vi "Cable Length Param.vi"(8 "error constant":errorcluster) -> (0 "error out":errorcluster, 2 "Cable Length Param":string)   [LabVIEW 2017]
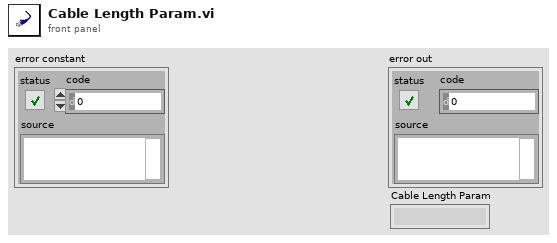
[diagram p1: front panel]
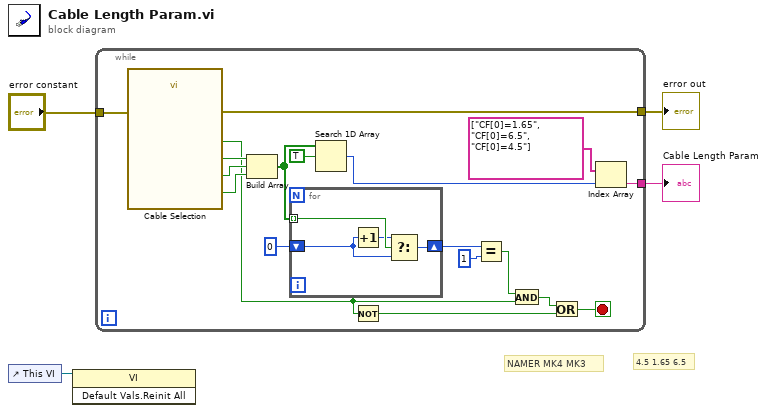
[diagram p0: block diagram]
diagram:
  # "4.5 1.65 6.5"
  # "NAMER MK4 MK3"
  n1 = control-ref of="This VI"() -> (w1:refnum<vi>)
  n2 = invoke class="VI" method="Default Vals.Reinit All"(reference=w1) -> ()  [unwired: 2 in, 3 out]
  n3 = while {
    tunnel: "error constant" -> [w20]
    tunnel: [w19] -> w3
    tunnel: [w9] -> w2
    stop <- w8 stop-if-true
    n4 = call "Cable Selection"("error in (no error)"=w20) -> ("NAMER"=w12:bool, "MK3"=w22:bool, "MK4"=w13:bool, "OK"=w5:bool, "error out"=w19:errorcluster)  [unwired: 14 in]
    n5 = Build Array(w13, w22, w12) -> (w18:bool[])
    n6 = for {
      tunnel: w18 -> [w26] mode=indexing
      shift-right: [w24] -> w16
      shift-left: 0 -> [w23]
      n7 = Increment(x=w23) -> (x+1=w25:i32)
      n8 = Select(t=w25, s=w26, f=w23) -> (s? t:f=w24:i32)
    }
    n9 = Search 1D Array(1D array=w18, element=TRUE) -> (index of element=w10:i32)  [unwired: 1 in]
    n10 = Not(x=w5) -> (.not. x?=w6:bool)
    n11 = Equal?(x=w16, y=1) -> (x = y?=w14:bool)
    n12 = And(x=w14, y=w5) -> (x .and. y?=w7:bool)
    n13 = Or(x=w7, y=w6) -> (x .or. y?=w8:bool)
    n14 = Index Array(array=string[] ["CF[0]=1.65", "CF[0]=6.5", "CF[0]=4.5"], index=w10) -> (element=w9:string)
  }
  "error out" <- w3
  "Cable Length Param" <- w2
